vi "pllot_text_side_cutting_offset.vi"(10 "D cutting offset array":ext[](array[numeric]), 11 "precision":i32) -> (0 "Left side length":string, 1 "Bottom side length":string, 2 "Right side length":string, 3 "Top side length":string)   [LabVIEW 2017]
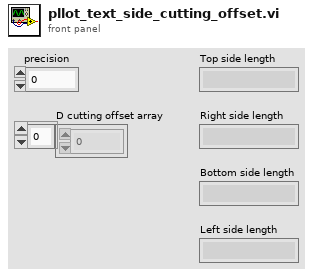
[diagram p1: front panel]
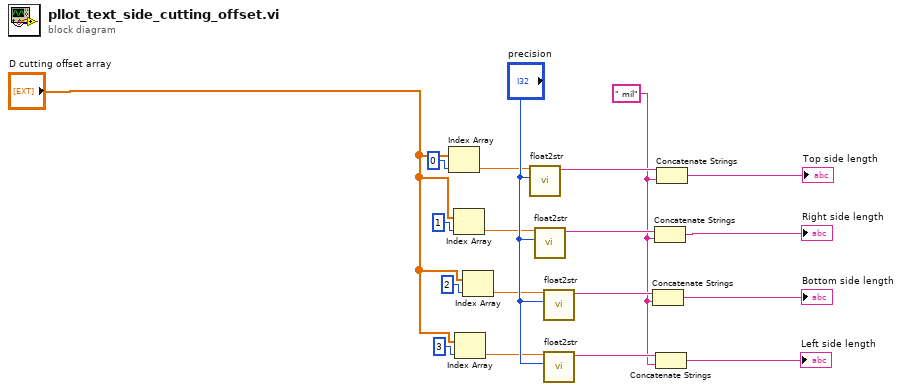
[diagram p0: block diagram]
diagram:
  w1 = " mil"
  n1 = Index Array(array="D cutting offset array", index=0) -> (element=w11:ext)
  n2 = Index Array(array="D cutting offset array", index=1) -> (element=w16:ext)
  n3 = Index Array(array="D cutting offset array", index=3) -> (element=w18:ext)
  n4 = Index Array(array="D cutting offset array", index=2) -> (element=w17:ext)
  n5 = call "float2str.vi"("precision"="precision", "float"=w11) -> ("string"=w9:string)  [unwired: 9 in]
  n6 = call "float2str.vi"("precision"="precision", "float"=w16) -> ("string"=w7:string)  [unwired: 9 in]
  n7 = call "float2str.vi"("precision"="precision", "float"=w17) -> ("string"=w5:string)  [unwired: 9 in]
  n8 = call "float2str.vi"("precision"="precision", "float"=w18) -> ("string"=w4:string)  [unwired: 9 in]
  n9 = Concatenate Strings(w5, w1) -> (→"Bottom side length":string)
  n10 = Concatenate Strings(w7, w1) -> (→"Right side length":string)
  n11 = Concatenate Strings(w4, w1) -> (→"Left side length":string)
  n12 = Concatenate Strings(w9, w1) -> (→"Top side length":string)
